vi "Request Data.vi"(4 "Ignore Past Updates? (F)":bool, 5 "Return Priority (Normal)":T1=enum."Normal", 6 "Value Changes Only? (T)":bool=TRUE, 8 "error in (no error)":errorcluster, 9 "Data Type":variant, 10 "Datum Name":string, 11 "IObserver in":refnum<class "IObserver.lvclass">) -> (0 "error out":errorcluster, 3 "IObserver out":refnum<class "IObserver.lvclass">)   [LabVIEW 2015, in "IObserver.lvlib" / "IObserver.lvclass"]
doc: "<License>\nCopyright © 2017 Composed Systems, LLC | All rights reserved\nwww.composed.io\n\nAuthor: Ethan Stern <ethan.stern@composed.io>\n\nThis software is provided \"AS IS\" WITHOUT WARRANTIES, either express or implied, AND IS FOR EDUCATIONAL PURPOSES ONLY.\n</License>"
uses:
  IObserver.lvclass
  <vilib>/ActorFramework/Message Enqueuer/Message Priority.ctl
  <vilib>/ActorFramework/Actor/Actor.lvclass/Actor.ctl
  <vilib>/ActorFramework/Message Enqueuer/Message Enqueuer.lvclass/Message Enqueuer.ctl
  IMediator/ISubscriptionPolicy/ISubscriptionPolicy.lvclass
  SubscriptionPolicy/ValueChangeSubscription/ValueChangeSubscription.lvclass/ValueChangeSubscription.ctl
  IObserver Messages/Subscribe Msg/Subscribe Msg.lvclass/Subscribe Msg.ctl
  <vilib>/ActorFramework/Message Enqueuer/Init from Existing Queue.vi
  <vilib>/ActorFramework/Message Enqueuer/Enqueue.vi
  <vilib>/ActorFramework/Message Priority Queue/Priority Enqueue.vi
  <vilib>/ActorFramework/Message Enqueuer/Message Enqueuer.lvclass
  SubscriptionPolicy/ValueChangeSubscription/ValueChangeSubscription.lvclass
  IObserver Messages/Subscribe Msg/Subscribe Msg.lvclass
  IMediator/SubscriptionRequest/SubscriptionRequest.lvclass
  <vilib>/ActorFramework/Actor/Actor.lvclass
  ActorDataBinding/ActorDataBinding.lvclass
panel:
  # "The idea of observing all data (not just value change)\nsmells like misuse of this portion of the API. If data\ntriggers action, use Notification Msg (ActorMessage\nTransport type)"
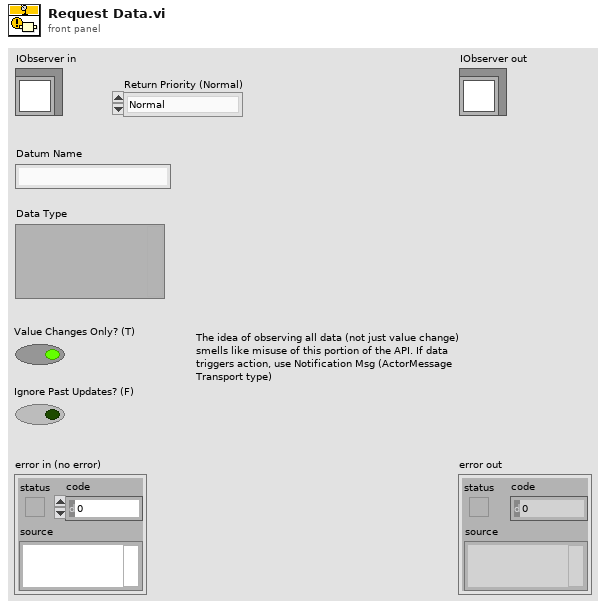
[diagram p1: front panel]
types:
  T1 = typedef "Actor Framework.lvlib/Message Enqueuer.lvclass/Message Priority.ctl" = enum16{"Low", "Normal", "High"}
  T2 = typedef "IMediator.lvlib/ISubscriptionPolicy.lvclass/ISubscriptionPolicy Reference.ctl" = refnum<data-value>
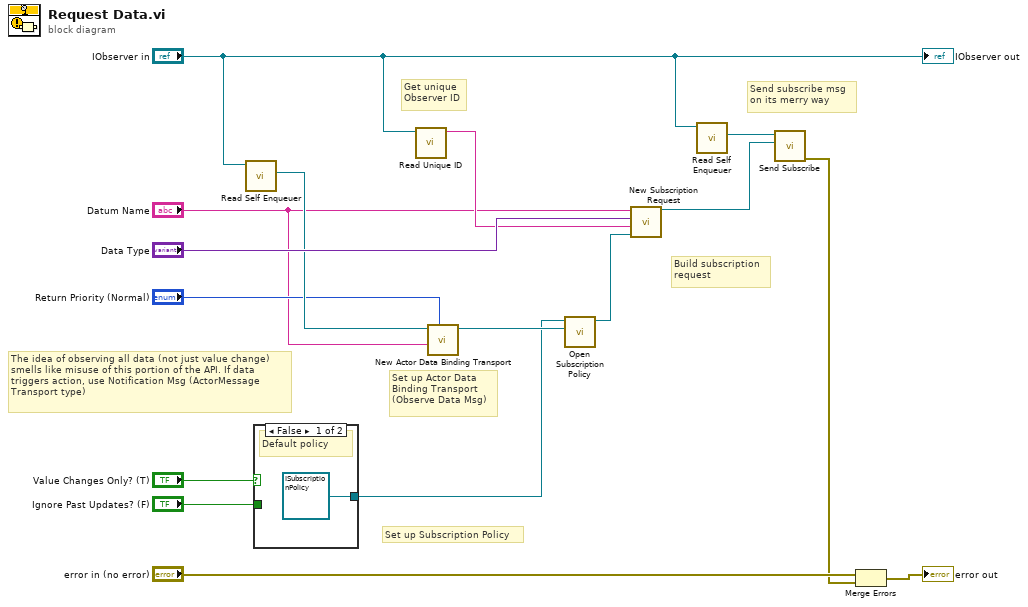
[diagram p0: block diagram]
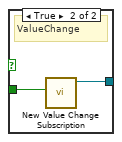
[diagram p2: hidden frame]
diagram:
  # "The idea of observing all data (not just value change)\nsmells like misuse of this portion of the API. If data\ntriggers action, use Notification Msg (ActorMessage\nTransport type)"
  # "Set up Subscription Policy"
  # "Send subscribe msg\non its merry way"
  # "Build subscription\nrequest"
  # "Get unique\nObserver ID"
  # "Set up Actor Data\nBinding Transport\n(Observe Data Msg)"
  n1 = call <vilib>:"Read Self Enqueuer.vi"("Actor"="IObserver in") -> ("Self Enqueuer"=w3:refnum<class "Message Enqueuer.lvclass">)  [unwired: 10 in]
  n2 = case shown="False" "Value Changes Only? (T)" {
    tunnel: "Ignore Past Updates? (F)" -> [_ w19]
    tunnel: [refnum<class "ISubscriptionPolicy.lvclass"> refnum ("IMediator.lvlib:ISubscriptionPolicy.lvclass") w18] -> w4
    frame False {
      # "Default policy"
    }
    frame True {
      # "ValueChange"
      n3 = call "New Value Change Subscription.vi"("Ignore Past Updates? (F)"=w19) -> ("ValueChangeSubscription Out"=w18:refnum<class "ValueChangeSubscription.lvclass">)  [unwired: 10 in]
    }
  }
  n4 = call "Read Unique ID.vi"("IObserver In"="IObserver in") -> ("Unique ID"=w9:string)  [unwired: 10 in]
  n5 = call "New Actor Data Binding Transport.vi"("Priority (Normal)"="Return Priority (Normal)", "Datum Return Name"="Datum Name", "IObserver"=w3) -> ("ActorDataBinding out"=w7:refnum<class "ActorDataBinding.lvclass">)  [unwired: 7 in, 1 out]
  n6 = call "Open Subscription Policy.vi"("Transport"=w7, "SubscriptionPolicy"=w4) -> ("Subscription Policy"=w8:T2)  [unwired: 8 in, 1 out]
  n7 = call "New Subscription Request.vi"("Subscription Policy"=w8, "Unique Subscriber ID"=w9, "Type"="Data Type", "Datum Name"="Datum Name") -> ("SubscriptionRequest"=w14:refnum<class "SubscriptionRequest.lvclass">)  [unwired: 7 in]
  n8 = call <vilib>:"Read Self Enqueuer.vi"("Actor"="IObserver in") -> ("Self Enqueuer"=w15:refnum<class "Message Enqueuer.lvclass">)  [unwired: 10 in]
  n9 = call "Send Subscribe.vi"("SubscriptionRequest"=w14, "Message Enqueuer"=w15) -> ("error out"=w12:errorcluster)  [unwired: 8 in, 1 out]
  n10 = Merge Errors("error in (no error)", w12) -> (→"error out":errorcluster)
  "IObserver out" <- "IObserver in"
